vi "Send custom move to stage.vi"(7 "Z pos":dbl[unit], 8 "error in (no error)":errorcluster, 9 "Y pos":dbl[unit], 10 "X pos":dbl[unit], 11 "Tomo in":refnum<class "Tomo.lvclass">) -> (0 "error out":errorcluster, 3 "Tomo out":refnum<class "Tomo.lvclass">)   [LabVIEW 2012, in "Tomo.lvclass"]
uses:
  Tomo.lvclass
  <vilib>/Distrio/Murmex/GenericMessage/GenericMessage.lvclass
  <vilib>/Distrio/Murmex/StartMessage/StartMessage.lvclass
  <vilib>/Distrio/Murmex/Message/Message.lvclass
  <vilib>/Distrio/Murmex/Murmex/Murmex.lvclass
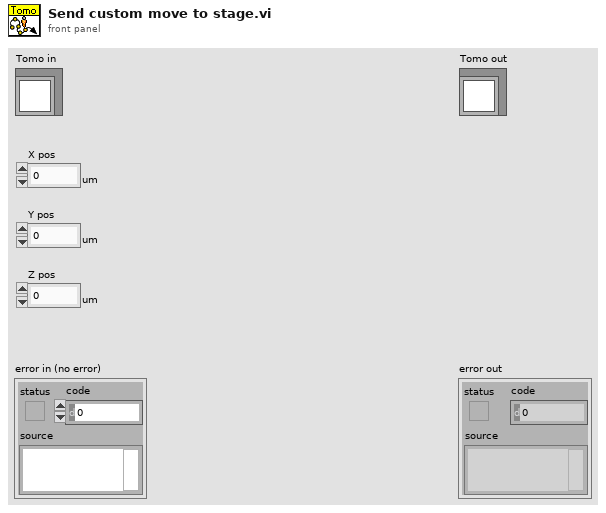
[diagram p1: front panel]
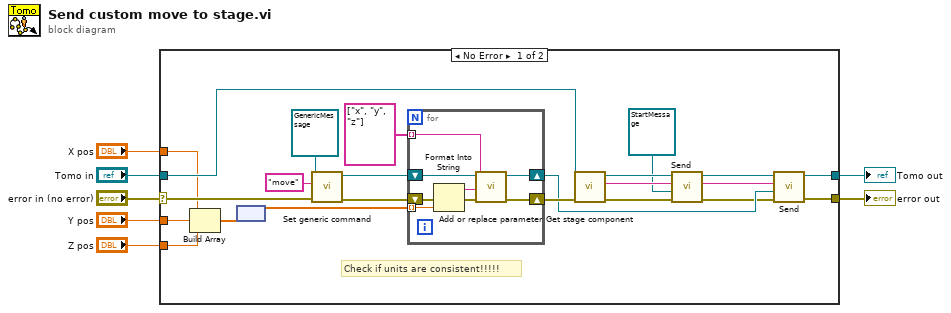
[diagram p0: block diagram]
diagram:
  n1 = case shown="No Error" "error in (no error)" {
    selector: "error in (no error)" -> [w14 w39]
    tunnel: [w13 w39] -> w6
    tunnel: [w11 w38] -> w4
    tunnel: "Tomo in" -> [w12 w38]
    tunnel: "X pos" -> [w10 _]
    tunnel: "Y pos" -> [w9 _]
    tunnel: "Z pos" -> [w8 _]
    frame No Error {
      # "Check if units are consistent!!!!!"
      n2 = Build Array(w10, w9, w8) -> (w24:dbl[unit][])
      n3 = node(w24) -> (w21:dbl[])
      n4 = call <vilib>:"Set generic command.vi"("error in (no error)"=w14, "generic command"="move" ("command string"), "GenericMessage in"=refnum<class "GenericMessage.lvclass"> refnum ("Murmex.lvlib:GenericMessage")) -> ("error out"=w27:errorcluster, "GenericMessage out"=w26:refnum<class "GenericMessage.lvclass">)  [unwired: 7 in]
      n5 = for {
        shift-right: [w31] -> w23
        shift-left: w27 -> [w37]
        shift-right: [w32] -> w22
        shift-left: w26 -> [w36]
        tunnel: string[] ["x", "y", "z"] -> [w34] mode=indexing
        tunnel: w21 -> [w33] mode=indexing
        n6 = Format Into String(error in=w37, w33) -> (resulting string=w30:string, error out=w35:errorcluster)  [unwired: 2 in]
        n7 = call <vilib>:"Add or replace parameter.vi"("error in (no error)"=w35, "value"=w30, "name"=w34, "Message in"=w36) -> ("error out"=w31:errorcluster, "Message out"=w32:refnum<class "GenericMessage.lvclass">)  [unwired: 6 in]
      }
      n8 = call-dynamic "Get stage component.vi"("error in (no error)"=w23, "Tomo in"=w12) -> ("error out"=w20:errorcluster, "stage component"=w16:string, "Tomo out"=w18:refnum<class "Tomo.lvclass">)  [unwired: 7 in]
      n9 = call <vilib>:"Send.vi"("error in (no error)"=w20, "Message"=refnum<class "StartMessage.lvclass"> refnum ("Distrio Murmex 1.1:StartMessage"), "recipient"=w16, "Murmex in"=w18) -> ("error out"=w19:errorcluster, "Murmex out"=w17:refnum<class "Tomo.lvclass">)  [unwired: 6 in]
      n10 = call <vilib>:"Send.vi"("error in (no error)"=w19, "Message"=w22, "recipient"=w16, "Murmex in"=w17) -> ("error out"=w13:errorcluster, "Murmex out"=w11:refnum<class "Tomo.lvclass">)  [unwired: 6 in]
    }
    frame Error {
    }
  }
  "error out" <- w6
  "Tomo out" <- w4
